vi "三转换ROI对比.vi"() -> ()   [LabVIEW 2018]
uses:
  <vilib>/vision/NI_Vision_Development_Module.lvlib
panel:
  out "Image 3":T1(plugin-control)
  out "Image 2":T1(plugin-control)
  out "error out":errorcluster
  out "元素":T2 {"Contours"."Type" items=["No Selection", "Point", "Line", "Rectangle", "Oval", "Polygon", "Freehand Region", "Annulus", "Unused2", "Unused3", "Broken Line", "Freehand Line", "Rotated Rectangle"]}
  in  "索引":i32
  out "Image":T1(plugin-control)
  in  "路径":path
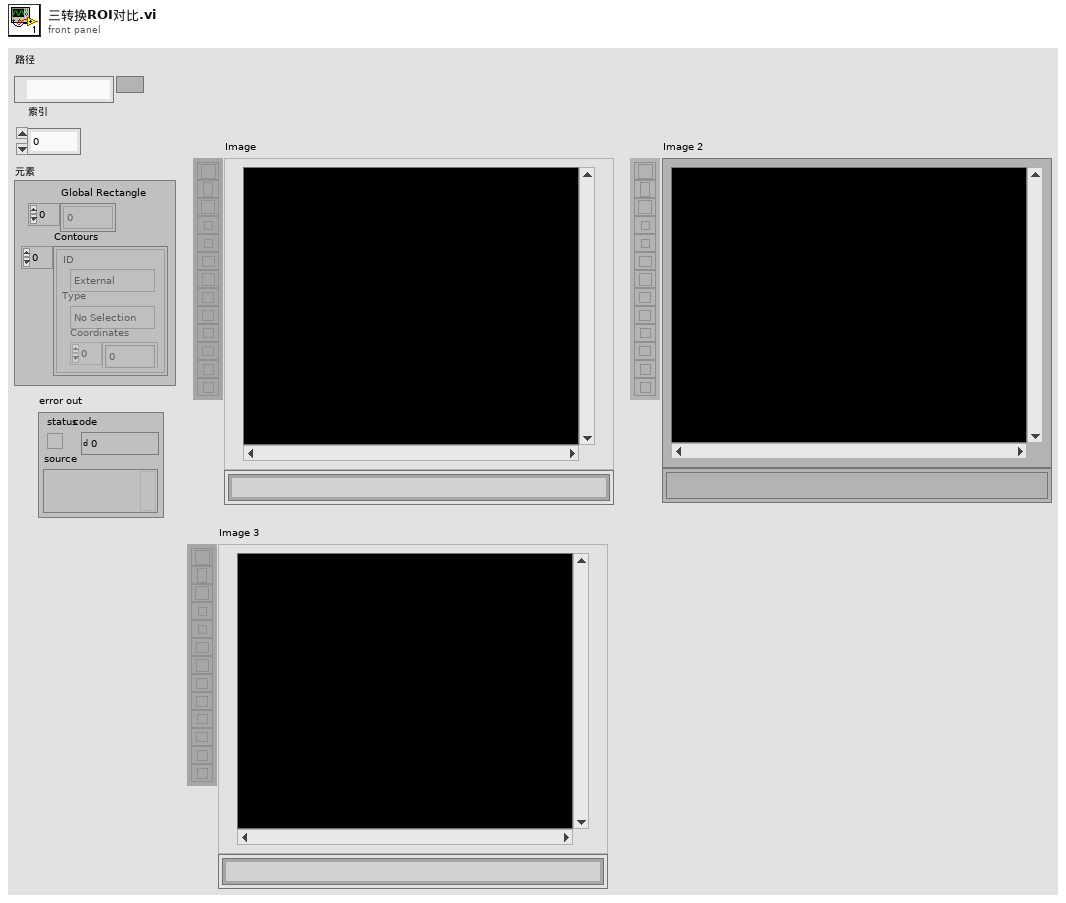
[diagram p1: front panel]
types:
  T1 = typedef "IMAQ Image.ctl" = refnum<image>
  T2 = typedef "ROI Descriptor" = cluster{"Global Rectangle":i32[], "Contours":cluster{"ID":enum32{"External", "Internal"}, "Type":u32, "Coordinates":i32[]}[]}
  T3 = typedef "Image Type" = u32
  T4 = cluster{"ID":enum32{"External", "Internal"}, "Type":u32, "Coordinates":i32[]}[]
  T5 = cluster{"ID":enum32{"External", "Internal"}, "Type":u32, "Coordinates":i32[]}
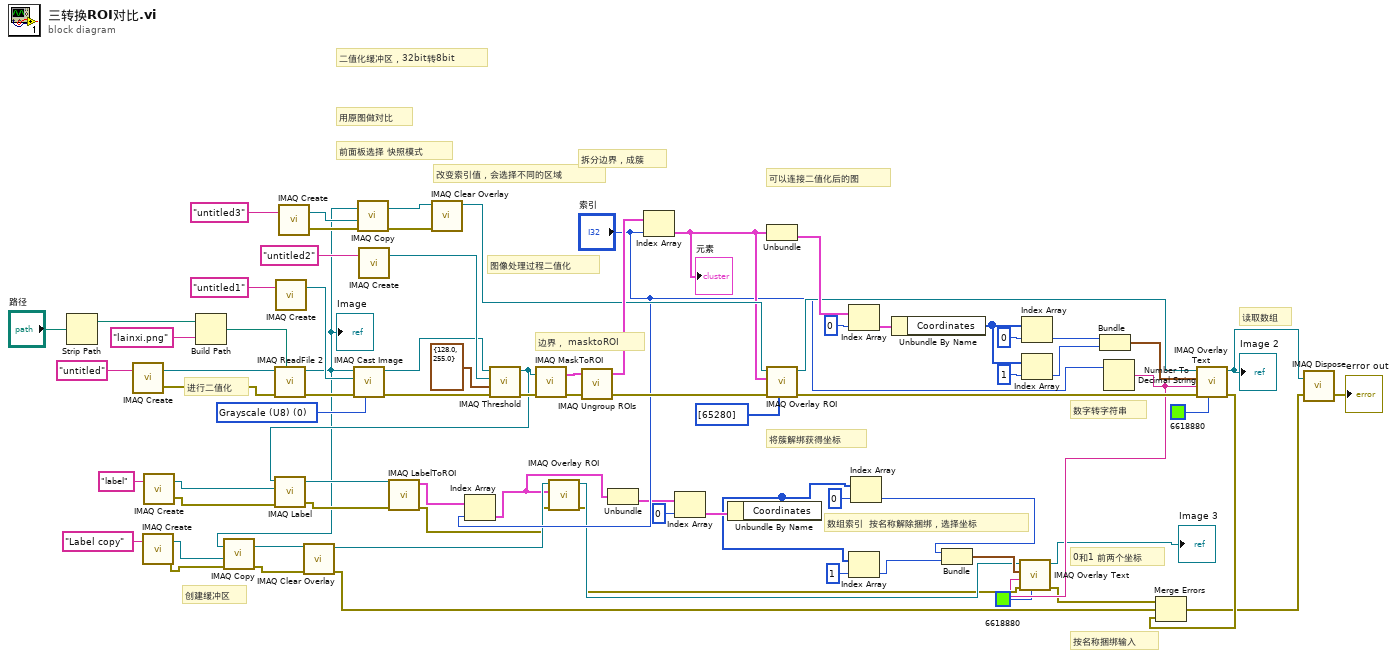
[diagram p0: block diagram]
diagram:
  w69 = T3 0 items=["Grayscale (U8)", "Grayscale (I16)", "Grayscale (SGL)", "Complex (CSG)", "RGB (U32)", "HSL (U32)", "RGB (U64)", "Grayscale (U16)"] ("Image Type")
  # "创建缓冲区"
  # "改变索引值，会选择不同的区域"
  # "前面板选择 快照模式"
  # "按名称捆绑输入"
  # "读取数组"
  # "0和1 前两个坐标"
  # "数组索引  按名称解除捆绑，选择坐标"
  # "将簇解绑获得坐标"
  # "数字转字符串"
  # "可以连接二值化后的图"
  # "用原图做对比"
  # "拆分边界，成簇"
  # "边界， masktoROI"
  # "图像处理过程二值化"
  # "二值化缓冲区，32bit转8bit"
  # "进行二值化"
  n1 = Strip Path(path="路径") -> (stripped path=w77:path)  [unwired: 1 out]
  n2 = call "IMAQ Create"("Image Name"="untitled") -> ("New Image"=w74:T1, "error out"=w73:errorcluster)  [unwired: 4 in]
  n3 = call "IMAQ Create"("Image Name"="Label copy") -> ("New Image"=w27:T1, "error out"=w24:errorcluster)  [unwired: 4 in]
  n4 = call "IMAQ Create"("Image Name"="label") -> ("New Image"=w34:T1, "error out"=w33:errorcluster)  [unwired: 4 in]
  n5 = Build Path(base path=w77, name or relative path="lainxi.png" ("名称或相对路径")) -> (appended path=w75:path)
  n6 = call "IMAQ ReadFile 2"("File Path"=w75, "error in (no error)"=w73, "Image"=w74) -> ("error out"=w68:errorcluster, "Image Out"=w26:T1)  [unwired: 4 in, 3 out]
  "Image" <- w26
  n7 = call "IMAQ Copy"("error in (no error)"=w24, "Image Dst"=w27, "Image Src"=w26) -> ("error out"=w22:errorcluster, "Image Dst Out"=w23:T1)  [unwired: 3 in]
  n8 = call "IMAQ Create"("Image Name"="untitled1") -> ("New Image"=w70:T1)  [unwired: 4 in, 1 out]
  n9 = call "IMAQ Create"("Image Name"="untitled3") -> ("New Image"=w56:T1, "error out"=w55:errorcluster)  [unwired: 4 in]
  n10 = call "IMAQ Clear Overlay"("error in (no error)"=w22, "Image"=w23) -> ("error out"=w5:errorcluster, "Image Out"=w21:T1)  [unwired: 8 in]
  n11 = call "IMAQ Cast Image"("Image Type"=w69, "error in (no error)"=w68, "Image Dst"=w70, "Image Src"=w26) -> ("error out"=w64:errorcluster, "Image Dst Out"=w66:T1)  [unwired: 6 in]
  n12 = call "IMAQ Copy"("error in (no error)"=w55, "Image Dst"=w56, "Image Src"=w26) -> ("error out"=w53:errorcluster, "Image Dst Out"=w54:T1)  [unwired: 3 in]
  n13 = call "IMAQ Create"("Image Name"="untitled2") -> ("New Image"=w67:T1)  [unwired: 4 in, 1 out]
  n14 = call "IMAQ Clear Overlay"("error in (no error)"=w53, "Image"=w54) -> ("Image Out"=w52:T1)  [unwired: 8 in, 1 out]
  n15 = call "IMAQ Threshold"("error in (no error)"=w64, "Range"=cluster{"Lower value":sgl, "Upper value":sgl} {"Lower value"=128.0, "Upper value"=255.0}, "Image Dst"=w67, "Image Src"=w66) -> ("error out"=w62:errorcluster, "Image Dst Out"=w32:T1)  [unwired: 6 in]
  n16 = call "IMAQ Label"("error in (no error)"=w33, "Image Dst"=w34, "Image Src"=w32) -> ("error out"=w30:errorcluster, "Image Dst Out"=w31:T1)  [unwired: 1 in, 1 out]
  n17 = call "IMAQ LabelToROI"("error in (no error)"=w30, "Image"=w31) -> ("error out"=w20:errorcluster, "ROIs"=w29:T2[])  [unwired: 6 in, 2 out]
  n18 = Index Array(array=w29, index="索引") -> (element=w19:T2)
  n19 = call "IMAQ MaskToROI"("Image"=w32, "error in (no error)"=w62) -> ("ROI Descriptor"=w61:T2, "error out"=w60:errorcluster)  [unwired: 5 in, 1 out]
  n20 = call "IMAQ Overlay ROI"("error in (no error)"=w20, "ROI Descriptor"=w19, "Image"=w21) -> ("error out"=w8:errorcluster, "Image Out"=w9:T1)  [unwired: 7 in]
  n21 = call "IMAQ Ungroup ROIs"("error in (no error)"=w60, "ROI Descriptor"=w61) -> ("error out"=w58:errorcluster, "ROI Descriptors out"=w59:T2[])  [unwired: 2 in]
  n22 = Unbundle(w19) -> ("Contours"=w18:T4)  [unwired: 1 out]
  n23 = Index Array(array=w59, index="索引") -> (element=w51:T2)
  "元素" <- w51
  n24 = Index Array(array=w18, index=0 ("索引")) -> (element=w16:T5)
  n25 = Unbundle By Name(w16) -> ("Coordinates"=w13:i32[])
  n26 = Unbundle(w51) -> ("Contours"=w50:T4)  [unwired: 1 out]
  n27 = call "IMAQ Overlay ROI"("Colors (Green)"=u32[] [65280], "error in (no error)"=w58, "ROI Descriptor"=w51, "Image"=w52) -> ("error out"=w41:errorcluster, "Image Out"=w40:T1)  [unwired: 6 in]
  n28 = Index Array(array=w50, index=0 ("索引")) -> (element=w48:T5)
  n29 = Index Array(array=w13, index=1 ("索引")) -> (element=w11:i32)
  n30 = Index Array(array=w13, index=0 ("索引")) -> (element=w12:i32)
  n31 = Unbundle By Name(w48) -> ("Coordinates"=w45:i32[])
  n32 = Bundle(w12, w11) -> (w10:cluster{i32, i32})  [unwired: 1 in]
  n33 = Index Array(array=w45, index=0 ("索引")) -> (element=w44:i32)
  n34 = Index Array(array=w45, index=1 ("索引")) -> (element=w43:i32)
  n35 = Bundle(w44, w43) -> (w42:cluster{i32, i32})  [unwired: 1 in]
  n36 = Number To Decimal String(number="索引") -> (decimal integer string=w7:string)  [unwired: 1 in]
  n37 = call "IMAQ Overlay Text"("Text Color (black)"=u32 6618880, "error in (no error)"=w8, "String"=w7, "Origin"=w10, "Image"=w9) -> ("error out"=w6:errorcluster, "Image Out"=→"Image 3":T1)  [unwired: 5 in]
  n38 = call "IMAQ Overlay Text"("Text Color (black)"=u32 6618880, "error in (no error)"=w41, "String"=w7, "Origin"=w42, "Image"=w40) -> ("error out"=w4:errorcluster, "Image Out"=w38:T1)  [unwired: 5 in]
  "Image 2" <- w38
  n39 = Merge Errors(w6, w5, w4) -> (w3:errorcluster)
  n40 = call "IMAQ Dispose"("Image"=w38, "error in (no error)"=w3) -> ("error out"=→"error out":errorcluster)  [unwired: 4 in]
